vi "Main FPGA 5-axis for Candy Packaging.vi"() -> ()   [LabVIEW 2014]
uses:
  <vilib>/Motion/MotorControl/_s/nism.interpretControlRegister.stateTransition.ctl
  SubVIs/Pulse Trigger.ctl
  <vilib>/Platform/TimedLoop/XDataNode/timing_clust.ctl
  <vilib>/Platform/TimedLoop/XDataNode/nitl_modes.ctl
  <vilib>/Platform/TimedLoop/XDataNode/wakeup.ctl
  <vilib>/Motion/MotorControl/_s/nism.digitalInputs.portA.ctl
  <vilib>/rvi/Emulation/niFpgaGetClockAttributes.vi
  <vilib>/rvi/Emulation/niFpgaSctlEmulationGetInTimedLoop.vi
  <vilib>/rvi/Emulation/niFpgaEmulationReportErrorSimple.vi
  Global FPGA.vi
  <vilib>/Motion/MotorControl/_s/nism.interpretControlRegister.indexed.vi
  <vilib>/rvi/Emulation/niFpgaProcessEmulError.vi
  <vilib>/Motion/MotorControl/_s/nism.mdo.read.positionLoopSyncData.vi
  <vilib>/Motion/MotorControl/_s/nism.mdo.read.splineData.vi
  <vilib>/Motion/MotorControl/_s/nism.generateStatusRegister.indexed.vi
  <vilib>/rvi/Emulation/niFpgaCriticalErrorInLSC.vi
  <vilib>/Motion/MotorControl/_s/nism.splineInterpolation.fxp.3.index.vi
  <vilib>/Motion/MotorControl/_s/nism.mdo.handler.indexed.vi
  <vilib>/Motion/MotorControl/_s/nism.digitalFilter.indexed.vi
  <vilib>/Motion/MotorControl/_s/nism.interpretDIOControl.portA.multiple.vi
  <vilib>/Motion/MotorControl/_s/nism.generateDIOStatus.portA.indexed.2.vi
  <vilib>/rvi/eio/common/nirviEmuTemplateMethod_errors.vi
  <vilib>/Motion/SoftMotion/Synchronization/nism.rioScan.generateSyncScan.vi
  <vilib>/rvi/Emulation/niFpgaEmulationIsFPGAContextNoSignature.vi
  <vilib>/rvi/FIFO/Fifo_Resource/nirvififoEmulationSetSize.vi
  <vilib>/rvi/DataTransferAndStorage/Container/Common/niFpgaContainerGetUniqueNameForEmu.vi
  <vilib>/rvi/FIFO/Fifo_Resource/nirviFifoEmulationQueueMgr.vi
  <instcachedir>/0/nirviFifoEmulationQueueMgr_E5CAEC123FF24DC58D834DCA3CDAA9B5.lvgen/nirviFifoEmulationQueueMgr_E5CAEC123FF24DC58D834DCA3CDAA9B5_004.vi
  <vilib>/rvi/errors/niFpgaSetErrorForExecOnDevCompSimple.vi
  <vilib>/rvi/eio/common/nirviEmuReportErrorAndStop.vi
  <vilib>/rvi/FIFO/Fifo_Resource/nirvififoEmulationDetermineInputValidOut.vi
  <vilib>/rvi/FIFO/Fifo_Resource/nirvififoEmulationCreateLock.vi
  <vilib>/rvi/FIFO/Fifo_Resource/nirvififoEmulationObtainLock.vi
  <vilib>/rvi/FIFO/Fifo_Resource/nirvififoEmulationReleaseLock.vi
  <vilib>/rvi/occurrence/nirviWaitOnOccurrenceBase.vi
  <vilib>/rvi/errors/nirviReportUnexpectedCaseInternalError.vi
  <vilib>/rvi/errors/nirviReportUnexpectedCaseInternalError (U32).vi
  <vilib>/eio/EIONode/EIONode.xnode
  <vilib>/Platform/TimedLoop/XDataNode/XDataNode.xnode
  <vilib>/rvi/DataTransferAndStorage/Container/XNode/niFpgaContainer.xnode
  <vilib>/rvi/FIFO/Fifo_Resource/nirvififoEmulationClear.vi
  <vilib>/rvi/FIFO/Fifo_Resource/nirvififoEmulationGetNumberOfElementsToRead.vi
  <vilib>/rvi/FIFO/Fifo_Resource/nirvififoEmulationWrite.vi
  <vilib>/Motion/MotorControl/NI_SoftMotion_MotorControlIP.lvlib
  <vilib>/Platform/TimedLoop/XDataNode/XDNodeRunTimeDep.lvlib
  <vilib>/Motion/SoftMotion/Synchronization/NI_SoftMotion_Synchronization.lvlib
panel:
  in  "Mark Sensor Simulation":bool
  out "FIFO Elements to Read":u32
  in  "Use sim?":bool=TRUE
  out "Mod3/DIO0":bool
  out "TPeriod (ticks)":u32
  in  "TPulse (ticks)":i32=2000
  in  "Ta (ticks)":i32
  in  "Tb (ticks)":i32
  in  "Number of pulses (N)":i32=4
  out "FIFO Write Timed Out?":bool
  out "Remainder (ticks)":i32
  out "Processed Pulse":i32[](array[numeric])
  out "Ta Error":bool
  out "Tb Error":bool
  out "Tpulse Error":bool
  in  "Process Engine Mode":enum16{"Auto Calc Tpulse", "Auto Calc Tb"}(ring)
  in  "Reset?":bool
  in  "Clear FIFO":bool
  out "Reset Flag":bool
  in  "TDelay (ticks)":i32
  out "Process Engine State":T1
  out "Armed":bool
  in  "Axis 5 Mode":enum16{"No Sync", "Sync with Sensor"}(ring)
  in  "Sensor Sync DIR":bool
  out "FIFO Read Timed Out?":bool
  out "Time elapsed (ticks)":u32
  out "Toggle Iterations":u32
  in  "Home 5":bool
  in  "Home 4":bool
  in  "Home 3":bool
  in  "Home 2":bool
  in  "Home 1":bool
  out "Home Limits":bool[](array[boolean])
  out "Fwd Limits":bool[](array[boolean])
  out "Rev Limits":bool[](array[boolean])
  out "Axis Positions":fxp<+/-,64,32>[](array[numeric])
  in  "STEP or CW? (T=STEP)":bool
  out "Drive Enable":bool[](array[boolean])
  in  "Enable Watchdog":bool
  in  "Pet Watchdog":bool
  in  "Watchdog Timeout Period (ticks)":u64=40000000 format="%.0p"
  out "Watchdog Timed Out?":bool
  out "Time Since Last Pet":u64
  in  "Enable value":bool
  in  "Drive Enable override?":bool
  out "State":T2=enum."Start --> Initializing" caption="state transition"
  in  "Sync Value":bool
  in  "Sync Enable override?":bool
  in  "Invert direction?":bool
  out "Sync is Fault":bool
  out "Sync is Locked":bool
  in  "minimum pulse":u16=40
  # "Synchronization Loop"
  # "Control Status Loop"
  # "Notes: \n1. This VI provides the communication interface between the NI SoftMotion Engine and the LabVIEW FPGA Module. You must compile this VI for a specific FPGA target before use. After compiling, run the VI before running any of the Express VI examples. For information on moving this example to another FPGA target, refer to ni.com/info and enter info code fpgaex.\n\n2. Only use the Reset Axis button if you are unable to communicate with the axis by any other means. This button resets the device state machine and other VIs to a known state. After resetting the axis, switch the NI Scan Engine from Active Mode to Configuration Mode, then back to Active Mode, before attempting to enable the axis."
  # "(These two buttons \nare for testing\npurposes.)"
  # "(These two buttons \nare for testing\npurposes.)"
  # "Step/Direction Loop"
  # "Mark Sensor Sync Options"
  # "FIFO Check"
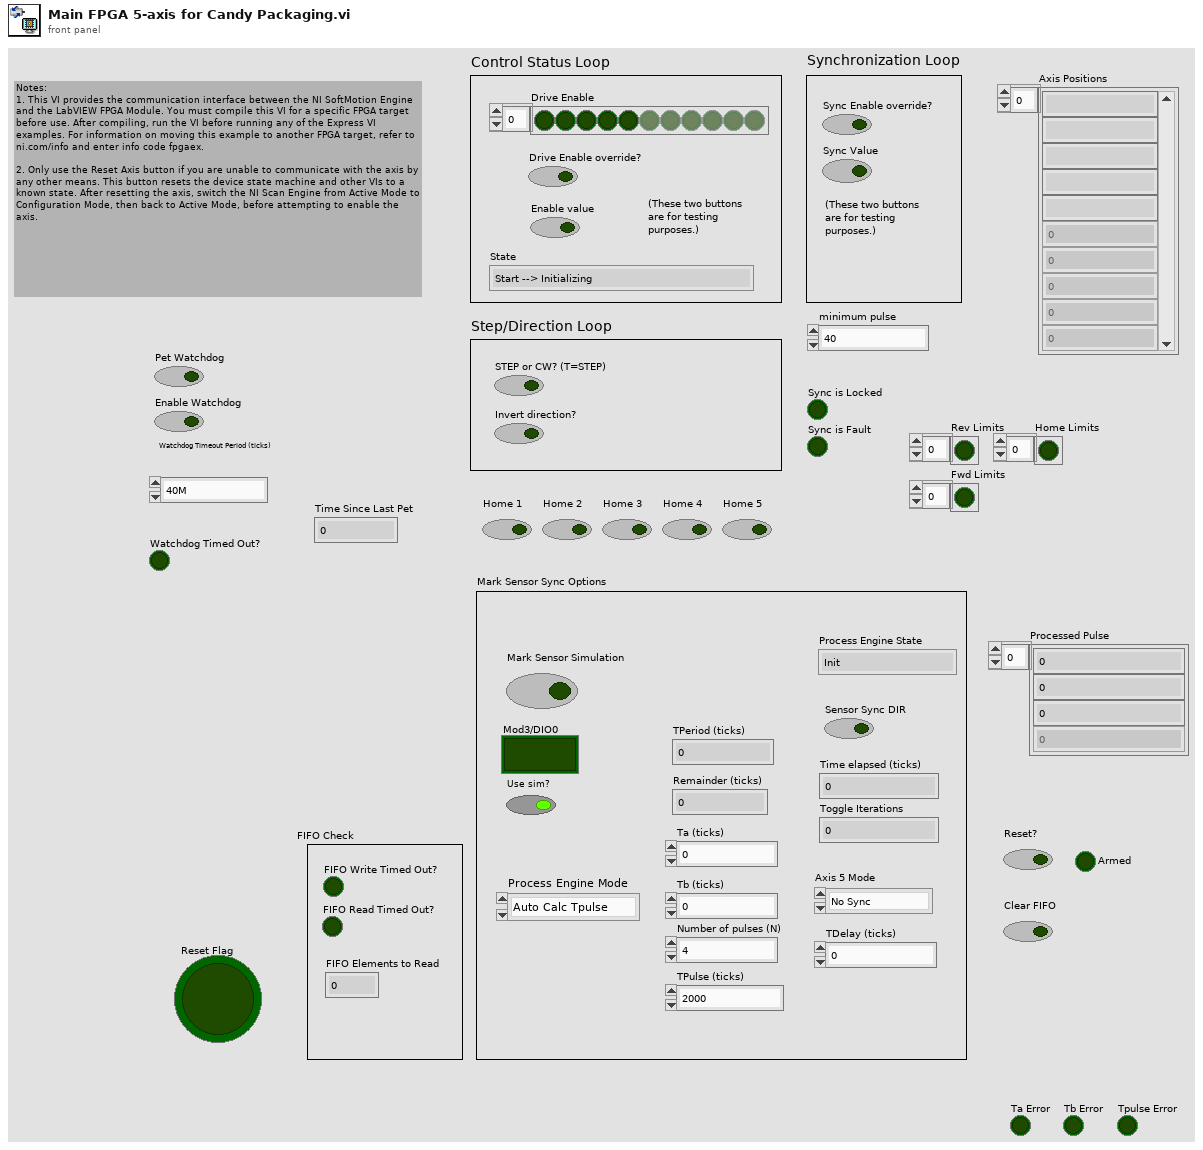
[diagram p1: front panel]
types:
  T1 = typedef "Pulse Trigger.ctl" = enum16{"Init", "Armed", "Processing"}
  T2 = typedef "NI_SoftMotion_MotorControlIP.lvlib/nism.interpretControlRegister.stateTransition.ctl" = enum8{"Invalid", "Start --> Initializing", "Initializing --> Disabled", "Disabled --> Ready To Switch On", "Ready To Switch On --> Switched On", "Ready To Switch On --> Disable", "Switched On --> Operation Enable", "Switched On --> Ready To Switch On", "Switched On --> Disabled", "Operation Enable --> Switched On", "Operation Enable --> Ready To Switch On", "Operation Enable --> Disabled", "Fault --> Disabled", "Any --> Fault", "None"}
  T3 = typedef "NI_SoftMotion_Synchronization.lvlib/nism.softmotionScan.timerConfig.ctl" = cluster{"target period (clocks)":u16, "host period / target period":u16}
  T4 = typedef "NI_SoftMotion_MotorControlIP.lvlib/nism.mdo.splineData.ctl" = cluster{"spline type":T5, "traj per/spline per":u16, "spline per/traj per":fxp<+,32,0>}
  T5 = typedef "NI_SoftMotion_MotorControlIP.lvlib/nism.splineInterpolation.type.ctl" = u16
  T6 = typedef "XDNodeRunTimeDep.lvlib/timing_clust.ctl" = cluster{"Expected End [f-1]":u64, "Actual End [f-1]":u64, "Finished Late? [f-1]":bool, "Expected End [i-1]":u64, "Actual End [i-1]":u64, "Finished Late? [i-1]":bool, "Expected Start [i]":u64, "Actual Start [i]":u64, "Expected Start [f]":u64, "Actual Start [f]":u64, "Source Name":string, "Structure Name":string, "Period":i64, "Deadline":i64, "Offset":i64, "Start":i64, "Priority":i32, "Timeout":i32, "Mode":T7, "Wakeup Reason":T8, "Error":errorcluster, "Source Type":string, "Secondary Source Type":string, "Global End Time":u64, "Global Start Time":u64, "Frame Duration":u64, "Iteration Duration":u64, "Assigned CPU":i32, "I/O Scan Engine Mode":u32}
  T7 = typedef "XDNodeRunTimeDep.lvlib/nitl_modes.ctl" = enum32{"No Change", "Process missed periods, maintain original phase", "Discard missed periods, maintain original phase", "Process missed periods, ignore original phase", "Discard missed periods, ignore original phase"}
  T8 = typedef "XDNodeRunTimeDep.lvlib/wakeup.ctl" = enum32{"Normal", "Aborted", "Asynchronous wakeup", "Timing source error", "Timed loop error", "Timeout"}
  T9 = typedef "NI_SoftMotion_Synchronization.lvlib/nism.softmotionScan.timerControl.ctl" = cluster{"sm scan":bool, "sm scan count":u32, "sm scan enabled":bool}
  T10 = typedef "NI_SoftMotion_MotorControlIP.lvlib/nism.digitalInputs.portA.ctl" = cluster{"reverse limit":bool, "forward limit":bool, "home switch":bool, "digital input 0":bool, "digital input 1":bool, "digital input 2":bool, "digital input 3":bool}
  T11 = typedef "NI_SoftMotion_MotorControlIP.lvlib/nism.dio.portA.config.2.ctl" = cluster{"digital filter (us)":u16[], "safe state":T12[]}
  T12 = typedef "nism.safeStates.ctl" = enum8{"Low", "High", "No Change"}
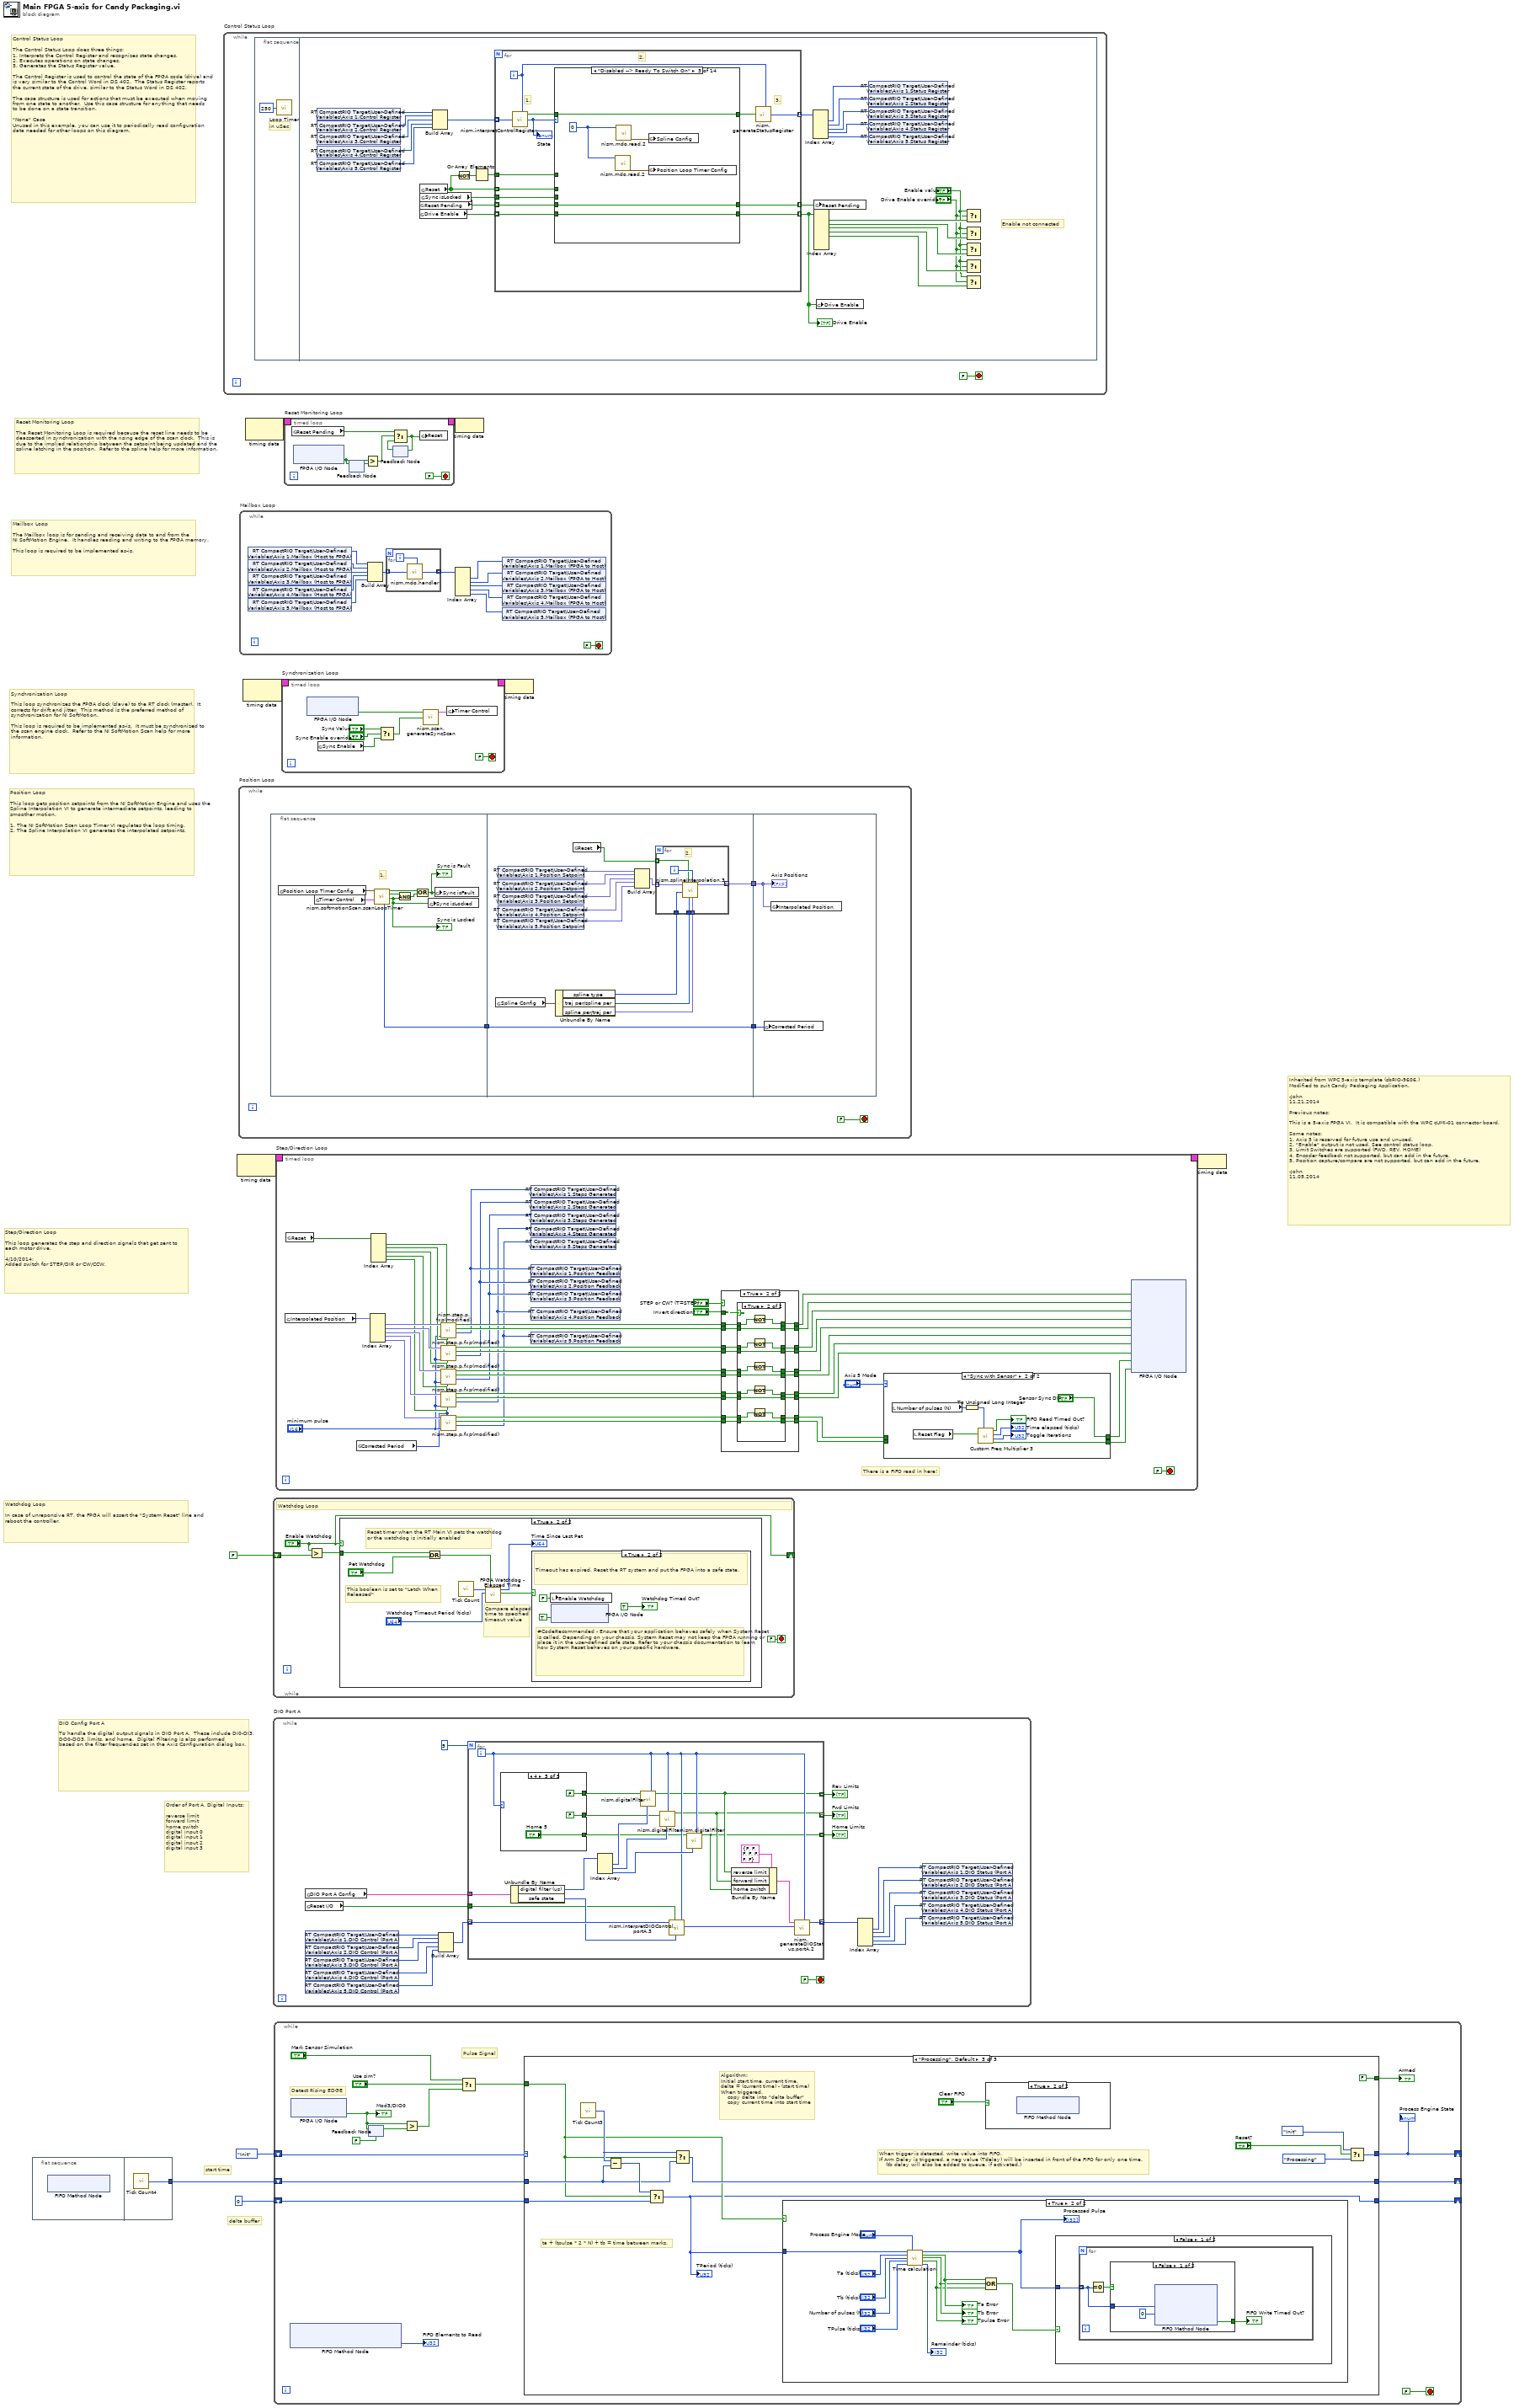
[diagram p0: block diagram]
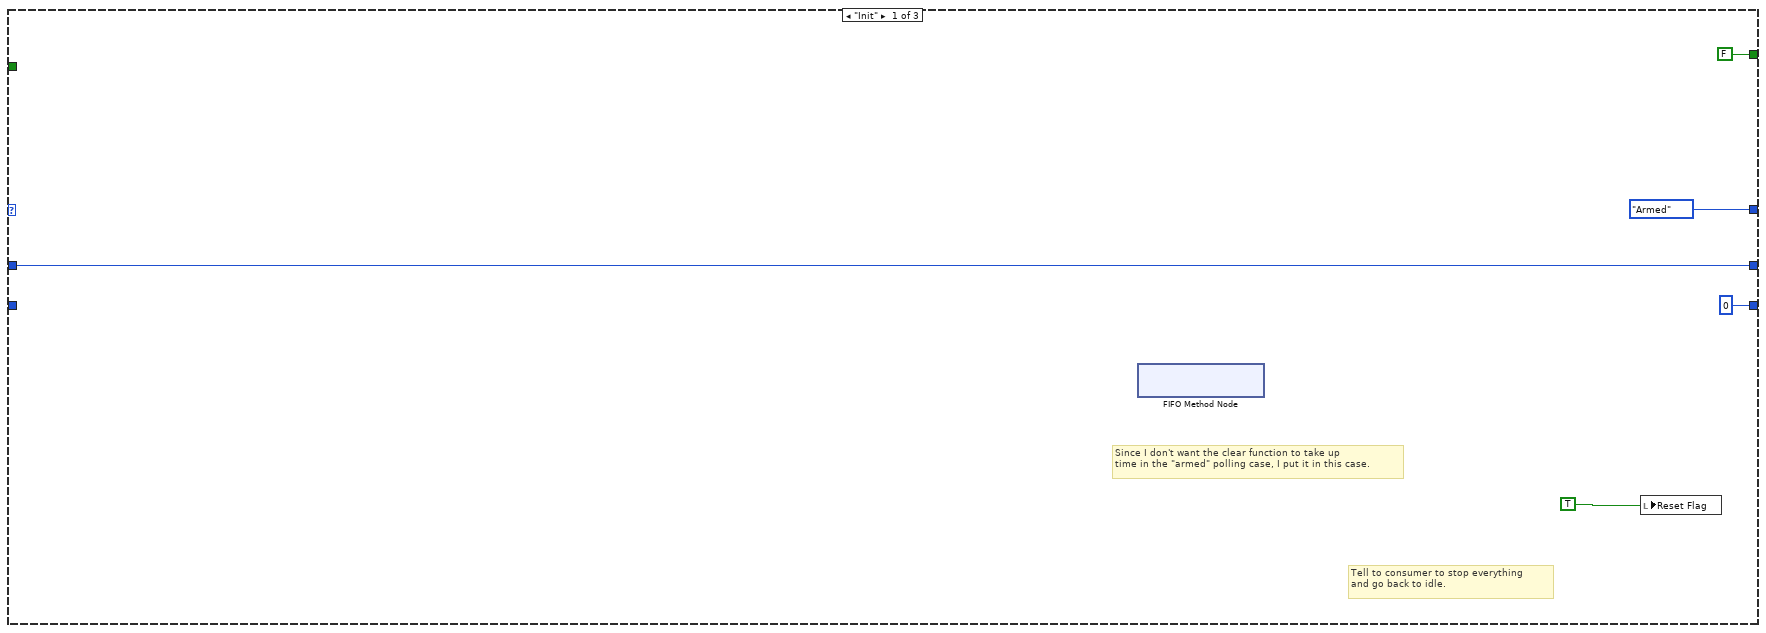
[diagram p2: hidden frame]
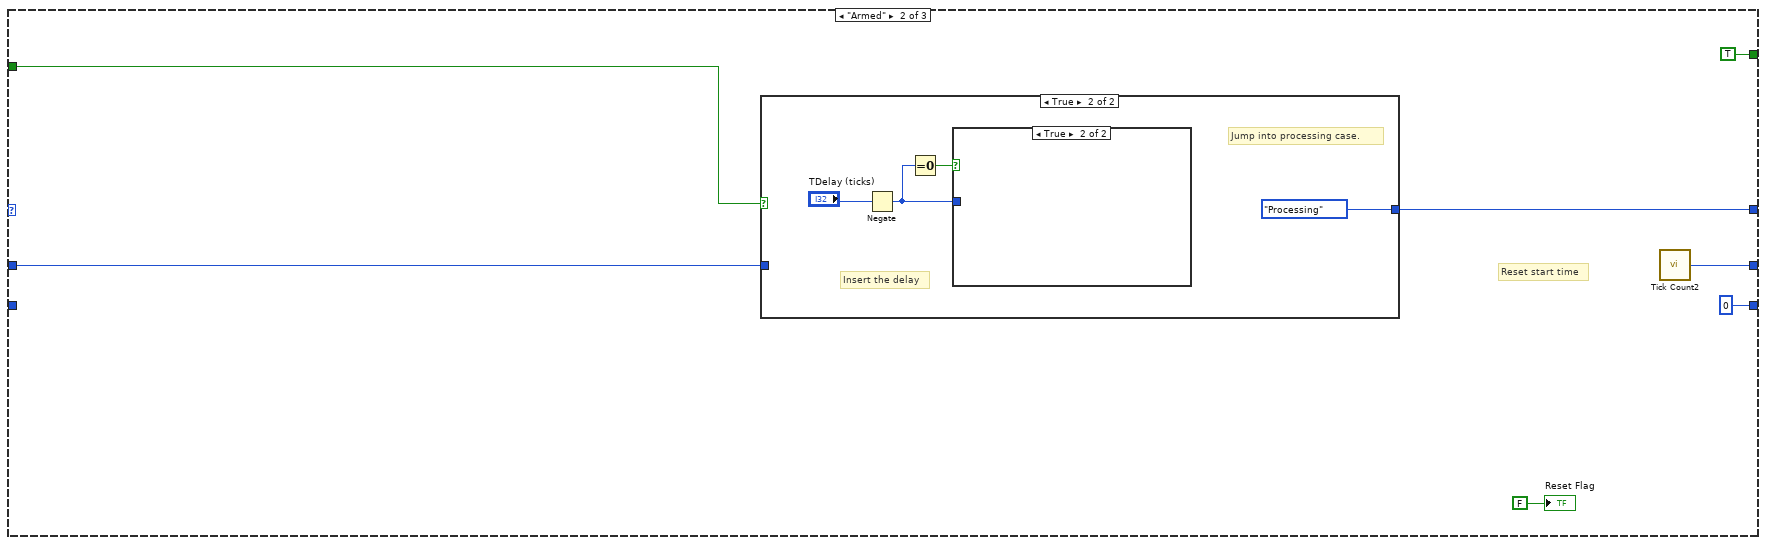
[diagram p3: hidden frame]
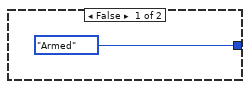
[diagram p4: hidden frame]
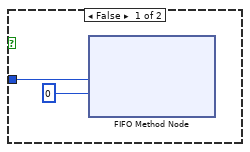
[diagram p5: hidden frame]
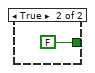
[diagram p8: hidden frame]
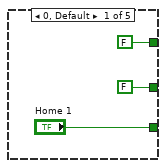
[diagram p10: hidden frame]
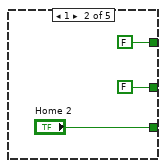
[diagram p11: hidden frame]
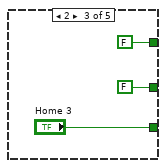
[diagram p12: hidden frame]
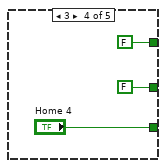
[diagram p13: hidden frame]
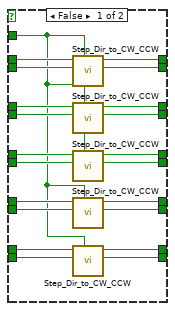
[diagram p17: hidden frame]
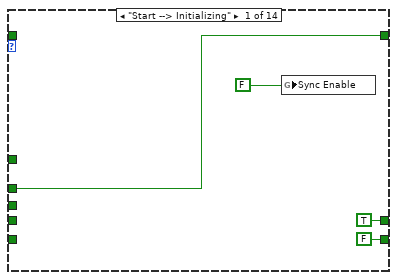
[diagram p19: hidden frame]
diagram:
  # "delta buffer"
  # "start time"
  # "Inherited from WPC 5-axis template (sbRIO-9606.)\nModified to suit Candy Packaging Application.\n\n-John\n11.21.2014\n\nPrevious notes:\n\nThis is a 5-axis FPGA VI.  It is compatible with the WPC cUMI-01 connector board.\n\nSome notes:\n1. Axis 5 is reserved for future use and unused.\n2. \"Enable\" output is not used. See control status loop.\n3. Limit Switches are supported (FWD, REV, HOME)\n4. Encoder feedback not supported, but can add in the future.\n5. Position capture/compare are not supported, but can add in the future.\n\n-John\n11.05.2014"
  # "DIO Config Port A\n\nTo handle the digital output signals in DIO Port A.  These include DI0-DI3, DO0-DO3, limits, and home.  Digital Filtering is also performed\nbased on the filter frequencies set in the Axis Configuration dialog box."
  # "Order of Port A, Digital Inputs:\n\nreverse limit\nforward limit\nhome switch\ndigital input 0\ndigital input 1\ndigital input 2\ndigital input 3"
  # "Watchdog Loop\n\nIn case of unreponsive RT, the FPGA will assert the \"System Reset\" line and reboot the controller."
  # "Step/Direction Loop\n\nThis loop generates the step and direction signals that get sent to \neach motor drive.\n\n4/10/2014:\nAdded switch for STEP/DIR or CW/CCW."
  # "Position Loop\n\nThis loop gets position setpoints from the NI SoftMotion Engine and uses the Spline Interpolation VI to generate intermediate setpoints, leading to smoother motion.\n\n1. The NI SoftMotion Scan Loop Timer VI regulates the loop timing. \n2. The Spline Interpolation VI generates the interpolated setpoints."
  # "Synchronization Loop\n\nThis loop synchronizes the FPGA clock (slave) to the RT clock (master).  It corrects for drift and jitter.  This method is the preferred method of synchronization for NI SoftMotion.\n\nThis loop is required to be implemented as-is.  It must be synchronized to the scan engine clock.  Refer to the NI SoftMotion Scan help for more information."
  # "Mailbox Loop\n\nThe Mailbox loop is for sending and receiving data to and from the \nNI SoftMotion Engine.  It handles reading and writing to the FPGA memory.\n\nThis loop is required to be implemented as-is."
  # "Reset Monitoring Loop\n\nThe Reset Monitoring Loop is required because the reset line needs to be deasserted in synchronization with the rising edge of the scan clock.  This is due to the implied relationship between the setpoint being updated and the spline latching in the position.  Refer to the spline help for more information."
  # "Control Status Loop\n\nThe Control Status Loop does three things:\n1. Interprets the Control Register and recognizes state changes.\n2. Executes operations on state changes.\n3. Generates the Status Register value.\n\nThe Control Register is used to control the state of the FPGA code (drive) and is very similar to the Control Word in DS 402.  The Status Register reports the current state of the drive, similar to the Status Word in DS 402.\n\nThe case structure is used for actions that must be executed when moving from one state to another.  Use this case structure for anything that needs to be done on a state transition.\n\n\"None\" Case\nUnused in this example, you can use it to periodically read configuration data needed for other loops on this diagram."
  n1 = flat-sequence {
    tunnel: [w11] -> w2
    frame #0 {
      n2 = xnode ("FIFO Method Node")() -> ()  [unwired: 1 in, 1 out]
    }
    frame #1 {
      n3 = call "Tick Count4"() -> ("Tick Count(Ticks)"=w11:u32)
    }
  }
  n4 = while "Control Status Loop" {
    stop <- FALSE stop-if-true
    n5 = flat-sequence {
      frame #0 {
        # "in uSec"
        n6 = call "Loop Timer"("Count(uSec)"=u32 250) -> ()  [unwired: 1 out]
      }
      frame #1 {
        # "Enable not connected"
        n7 = shared-variable "RT CompactRIO Target\\User-Defined Variables\\Axis 1.Control Register"() -> (w30:u32)  [unwired: 1 in, 1 out]
        n8 = shared-variable "RT CompactRIO Target\\User-Defined Variables\\Axis 2.Control Register"() -> (w29:u32)  [unwired: 1 in, 1 out]
        n9 = shared-variable "RT CompactRIO Target\\User-Defined Variables\\Axis 3.Control Register"() -> (w28:u32)  [unwired: 1 in, 1 out]
        n10 = shared-variable "RT CompactRIO Target\\User-Defined Variables\\Axis 4.Control Register"() -> (w27:u32)  [unwired: 1 in, 1 out]
        n11 = shared-variable "RT CompactRIO Target\\User-Defined Variables\\Axis 5.Control Register"() -> (w26:u32)  [unwired: 1 in, 1 out]
        n12 = global read "Global FPGA.vi" "Reset Pending"() -> (w34:bool[])
        n13 = global read "Global FPGA.vi" "Drive Enable"() -> (w33:bool[])
        n14 = global read "Global FPGA.vi" "Reset"() -> (w35:bool[])
        n15 = global read "Global FPGA.vi" "Sync isLocked"() -> (w40:bool)
        n16 = Build Array(w30, w29, w28, w27, w26) -> (w39:u32[])
        n17 = Not(x=w35) -> (.not. x?=w37:bool[])
        n18 = Or Array Elements(Boolean array=w37) -> (logical OR=w36:bool)
        n19 = for {
          tunnel: w35 -> [w48] mode=indexing
          tunnel: w40 -> [w47]
          tunnel: w39 -> [w49] mode=indexing
          tunnel: [w46] -> w31 mode=indexing
          tunnel: [w45] -> w38 mode=indexing
          tunnel: [w44] -> w32 mode=indexing
          tunnel: w36 -> [w43]
          tunnel: w34 -> [w42] mode=indexing
          tunnel: w33 -> [w41] mode=indexing
          i -> [w50]
          # "3."
          # "2."
          # "1."
          n20 = call-poly <vilib>:"nism.interpretControlRegister.vi"("control register"=w49, "axis index"=w50) -> ("transition occurred"=w51:bool, "state transition"=w52:T2)  [unwired: 6 in]
          "State" <- w52
          n21 = case shown="\"Disabled --> Ready To Switch On\"" w52 {
            tunnel: w51 -> [_ w60 w66 _ w73 _ w81 w85 _ _ _ _ w105 _]
            tunnel: [w57 w60 w66 w68 w73 w77 w81 w85 w87 w90 w94 w98 w104 _] -> w53
            tunnel: w48 -> [w57 _ _ _ _ w76 _ _ w87 w90 w94 w98 _ _]
            tunnel: w47 -> [_ _ _ w68 _ _ _ _ _ _ _ _ _ _]
            tunnel: [TRUE ("Write.Reset Pending") w59 w63 w67 w72 FALSE ("Write.Reset Pending") w78 w82 TRUE ("Write.Reset Pending") TRUE ("Write.Reset Pending") TRUE ("Write.Reset Pending") TRUE ("Write.Reset Pending") w102 w107] -> w45
            tunnel: [FALSE ("Write.Drive Enable") w58 w62 TRUE ("Write.Drive Enable") w71 w74 FALSE ("Write.Drive Enable") FALSE ("Write.Drive Enable") w86 FALSE ("Write.Drive Enable") FALSE ("Write.Drive Enable") FALSE ("Write.Drive Enable") w101 w106] -> w44
            tunnel: w43 -> [_ _ _ _ _ _ w79 w83 _ w89 w93 w97 w103 _]
            tunnel: w42 -> [_ w59 w63 w67 w72 _ w78 w82 _ _ _ _ w102 w107]
            tunnel: w41 -> [_ w58 w62 _ w71 w74 _ _ w86 _ _ _ w101 w106]
            frame "Start --> Initializing" {
              n22 = global write "Global FPGA.vi" "Sync Enable"(FALSE ("Sync Enable")) -> ()
            }
            frame "Initializing --> Disabled" {
            }
            frame "Disabled --> Ready To Switch On" {
              w61 = 0 ("axis index")
              n23 = call-poly <vilib>:"nism.mdo.read.2.vi"("axis index"=w61) -> ("position loop sync"=w64:T3)  [unwired: 10 in]
              n24 = call-poly <vilib>:"nism.mdo.read.2.vi"("axis index"=w61) -> ("spline"=w65:T4)  [unwired: 10 in]
              n25 = global write "Global FPGA.vi" "Spline Config"(w65) -> ()
              n26 = global write "Global FPGA.vi" "Position Loop Timer Config"(w64) -> ()
            }
            frame "Ready To Switch On --> Switched On" {
              n27 = global write "Global FPGA.vi" "Sync Enable"(TRUE ("Sync Enable")) -> ()
            }
            frame "Ready To Switch On --> Disable" {
            }
            frame "Switched On --> Operation Enable" {
              n28 = Not(x=w76) -> (.not. x?=w77:bool)
            }
            frame "Switched On --> Ready To Switch On" {
              n29 = global write "Global FPGA.vi" "Sync Enable"(w79) -> ()
            }
            frame "Switched On --> Disabled" {
              n30 = global write "Global FPGA.vi" "Sync Enable"(w83) -> ()
            }
            frame "Operation Enable --> Switched On" {
            }
            frame "Operation Enable --> Ready To Switch On" {
              n31 = global write "Global FPGA.vi" "Sync Enable"(w89) -> ()
            }
            frame "Operation Enable --> Disabled" {
              n32 = global write "Global FPGA.vi" "Sync Enable"(w93) -> ()
            }
            frame "Any --> Fault" {
              n33 = global write "Global FPGA.vi" "Sync Enable"(w97) -> ()
            }
            frame "Fault --> Disabled" {
              # "wait one cycle for clear faults to have taken effect"
              n34 = global write "Global FPGA.vi" "Sync Enable"(w103) -> ()
              n35 = Not(x=w105) -> (.not. x?=w104:bool)
            }
            frame "None", Default {
            }
          }
          n36 = call-poly <vilib>:"nism.generateStatusRegister.vi"("transition success"=w53, "axis index"=w50) -> ("status register"=w46:u32)  [unwired: 7 in]
        }
        "Drive Enable" <- w32
        n37 = Index Array(array=w31) -> (element #1=w25:u32, element #2=w24:u32, element #3=w23:u32, element #4=w22:u32, element #5=w21:u32)  [unwired: 5 in]
        n38 = global write "Global FPGA.vi" "Reset Pending"(w38) -> ()
        n39 = Index Array(array=w32) -> (element #1=w20:bool, element #2=w19:bool, element #3=w18:bool, element #4=w17:bool, element #5=w16:bool)  [unwired: 8 in, 3 out]
        n40 = global write "Global FPGA.vi" "Drive Enable"(w32) -> ()
        n41 = shared-variable "RT CompactRIO Target\\User-Defined Variables\\Axis 1.Status Register"(w25) -> ()  [unwired: 1 in, 1 out]
        n42 = shared-variable "RT CompactRIO Target\\User-Defined Variables\\Axis 2.Status Register"(w24) -> ()  [unwired: 1 in, 1 out]
        n43 = shared-variable "RT CompactRIO Target\\User-Defined Variables\\Axis 3.Status Register"(w23) -> ()  [unwired: 1 in, 1 out]
        n44 = shared-variable "RT CompactRIO Target\\User-Defined Variables\\Axis 4.Status Register"(w22) -> ()  [unwired: 1 in, 1 out]
        n45 = shared-variable "RT CompactRIO Target\\User-Defined Variables\\Axis 5.Status Register"(w21) -> ()  [unwired: 1 in, 1 out]
        n46 = Select(t="Enable value", s="Drive Enable override?", f=w20) -> ()  [unwired: 1 out]
        n47 = Select(t="Enable value", s="Drive Enable override?", f=w19) -> ()  [unwired: 1 out]
        n48 = Select(t="Enable value", s="Drive Enable override?", f=w18) -> ()  [unwired: 1 out]
        n49 = Select(t="Enable value", s="Drive Enable override?", f=w17) -> ()  [unwired: 1 out]
        n50 = Select(t="Enable value", s="Drive Enable override?", f=w16) -> ()  [unwired: 1 out]
      }
    }
  }
  n51 = node-c288() -> (w10:T6)  [unwired: 1 in]
  n52 = while "Position Loop" {
    stop <- FALSE stop-if-true
    n53 = flat-sequence {
      tunnel: [w112] -> w108
      tunnel: [w126] -> w110
      tunnel: [w125] -> w109
      tunnel: w108 -> [w125]
      tunnel: w110 -> [w140]
      tunnel: w109 -> [w141]
      frame #0 {
        # "1."
        n54 = global read "Global FPGA.vi" "Position Loop Timer Config"() -> (w114:T3)
        n55 = global read "Global FPGA.vi" "Timer Control"() -> (w113:T9)
        n56 = call <vilib>:"nism.softmotionScan.scanLoopTimer.vi"("timer control"=w113, "timer config"=w114) -> ("scan running?"=w116:bool, "finished late?"=w118:bool, "fault occurred?"=w119:bool, "corrected period"=w112:u16)  [unwired: 5 in, 1 out]
        "Sync is Locked" <- w116
        n57 = Compound Arithmetic op=AND(w118, w116) -> (w117:bool)
        n58 = Compound Arithmetic op=OR(w119, w117) -> (w115:bool)
        "Sync is Fault" <- w115
        n59 = global write "Global FPGA.vi" "Sync isLocked"(w116) -> ()
        n60 = global write "Global FPGA.vi" "Sync isFault"(w115) -> ()
      }
      frame #1 {
        n61 = global read "Global FPGA.vi" "Spline Config"() -> (w128:T4)
        n62 = shared-variable "RT CompactRIO Target\\User-Defined Variables\\Axis 1.Position Setpoint"() -> (w124:fxp<+/-,64,32>)  [unwired: 1 in, 1 out]
        n63 = shared-variable "RT CompactRIO Target\\User-Defined Variables\\Axis 2.Position Setpoint"() -> (w123:fxp<+/-,64,32>)  [unwired: 1 in, 1 out]
        n64 = shared-variable "RT CompactRIO Target\\User-Defined Variables\\Axis 3.Position Setpoint"() -> (w122:fxp<+/-,64,32>)  [unwired: 1 in, 1 out]
        n65 = shared-variable "RT CompactRIO Target\\User-Defined Variables\\Axis 4.Position Setpoint"() -> (w121:fxp<+/-,64,32>)  [unwired: 1 in, 1 out]
        n66 = shared-variable "RT CompactRIO Target\\User-Defined Variables\\Axis 5.Position Setpoint"() -> (w120:fxp<+/-,64,32>)  [unwired: 1 in, 1 out]
        n67 = Unbundle By Name(w128) -> ("spline type"=w132:T5, "traj per/spline per"=w131:u16, "spline per/traj per"=w130:fxp<+,32,0>)
        n68 = global read "Global FPGA.vi" "Reset"() -> (w127:bool[])
        n69 = Build Array(w124, w123, w122, w121, w120) -> (w129:fxp<+/-,64,32>[])
        n70 = for {
          tunnel: w132 -> [w139]
          tunnel: w131 -> [w138]
          tunnel: w130 -> [w137]
          tunnel: w127 -> [w134] mode=indexing
          tunnel: w129 -> [w136] mode=indexing
          tunnel: [w133] -> w126 mode=indexing
          i -> [w135]
          # "2."
          n71 = call-poly <vilib>:"nism.splineInterpolation.3.vi"("1 / calls per sample"=w137, "index"=w135, "calls per sample"=w138, "reset"=w134, "spline type"=w139, "x"=w136) -> ("xi"=w133:fxp<+/-,64,32>)  [unwired: 4 in, 1 out]
        }
      }
      frame #2 {
        n72 = global write "Global FPGA.vi" "Corrected Period"(w141) -> ()
        n73 = global write "Global FPGA.vi" "Interpolated Position"(w140) -> ()
        "Axis Positions" <- w140
      }
    }
  }
  n74 = while "Mailbox Loop" {
    stop <- FALSE stop-if-true
    n75 = shared-variable "RT CompactRIO Target\\User-Defined Variables\\Axis 1.Mailbox (Host to FPGA)"() -> (w151:u64)  [unwired: 1 in, 1 out]
    n76 = shared-variable "RT CompactRIO Target\\User-Defined Variables\\Axis 2.Mailbox (Host to FPGA)"() -> (w150:u64)  [unwired: 1 in, 1 out]
    n77 = shared-variable "RT CompactRIO Target\\User-Defined Variables\\Axis 3.Mailbox (Host to FPGA)"() -> (w149:u64)  [unwired: 1 in, 1 out]
    n78 = shared-variable "RT CompactRIO Target\\User-Defined Variables\\Axis 4.Mailbox (Host to FPGA)"() -> (w148:u64)  [unwired: 1 in, 1 out]
    n79 = shared-variable "RT CompactRIO Target\\User-Defined Variables\\Axis 5.Mailbox (Host to FPGA)"() -> (w147:u64)  [unwired: 1 in, 1 out]
    n80 = Build Array(w151, w150, w149, w148, w147) -> (w153:u64[])
    n81 = for {
      tunnel: w153 -> [w157] mode=indexing
      tunnel: [w156] -> w152 mode=indexing
      i -> [w155]
      n82 = call-poly <vilib>:"nism.mdo.handler.vi"("mbox (host to fpga)"=w157, "axis index"=w155) -> ("mbox (fpga to host)"=w156:u64)  [unwired: 7 in]
    }
    n83 = Index Array(array=w152) -> (element #1=w146:u64, element #2=w145:u64, element #3=w144:u64, element #4=w143:u64, element #5=w142:u64)  [unwired: 5 in]
    n84 = shared-variable "RT CompactRIO Target\\User-Defined Variables\\Axis 5.Mailbox (FPGA to Host)"(w142) -> ()  [unwired: 1 in, 1 out]
    n85 = shared-variable "RT CompactRIO Target\\User-Defined Variables\\Axis 1.Mailbox (FPGA to Host)"(w146) -> ()  [unwired: 1 in, 1 out]
    n86 = shared-variable "RT CompactRIO Target\\User-Defined Variables\\Axis 2.Mailbox (FPGA to Host)"(w145) -> ()  [unwired: 1 in, 1 out]
    n87 = shared-variable "RT CompactRIO Target\\User-Defined Variables\\Axis 3.Mailbox (FPGA to Host)"(w144) -> ()  [unwired: 1 in, 1 out]
    n88 = shared-variable "RT CompactRIO Target\\User-Defined Variables\\Axis 4.Mailbox (FPGA to Host)"(w143) -> ()  [unwired: 1 in, 1 out]
  }
  n89 = node-c288() -> (w8:T6)  [unwired: 1 in]
  n90 = node-c288() -> (w6:T6)  [unwired: 1 in]
  n91 = while "RT Watchdog Loop" {
    shift-right: ["Enable Watchdog"] -> _
    shift-left: FALSE ("Enable RT Watchdog") -> [w161]
    stop <- FALSE stop-if-true
    # "Watchdog Loop"
    n92 = Greater?(x="Enable Watchdog", y=w161) -> (0:w158:bool)
    n93 = case shown="True" "Enable Watchdog" {
      tunnel: w158 -> [_ w164]
      frame False {
        # "This loop has to be explicitly enabled from the RT Main VI.  This reduces the possiblity of an endless reboot cycle."
      }
      frame True {
        # "This boolean is set to \"Latch When Released\""
        # "Compare elapsed time to specified timeout value"
        # "Reset timer when the RT Main VI pets the watchdog or the watchdog is initially enabled"
        n94 = Or(x=w164, y="Pet Watchdog") -> (x .or. y?=w163:bool)
        n95 = call "Tick Count"() -> ("Tick Count(Ticks)"=w167:u32)
        n96 = call "FPGA Watchdog - Elapsed Time.vi"("Reset"=w163, "Timeout Period"="Watchdog Timeout Period (ticks)", "Current Time"=w167) -> ("Timeout"=w162:bool, "Elapsed Time"=→"Time Since Last Pet":u64)  [unwired: 7 in]
        n97 = case shown="True" w162 {
          frame False {
            # "Timeout has not expired."
          }
          frame True {
            # "#CodeRecommended - Ensure that your application behaves safely when System Reset is called. Depending on your chassis, System Reset may not keep the FPGA running or place it in the user-defined safe state. Refer to your chassis documentation to learn how System Reset behaves on your specific hardware."
            # "Timeout has expired. Reset the RT system and put the FPGA into a safe state."
            n98 = local write "Enable Watchdog"(FALSE ("Enable RT Watchdog")) -> ()
            n99 = xnode "FPGA I/O Node"("System Reset"=TRUE ("RT Reset on Watchdog Failure?")) -> ()  [unwired: 1 in, 1 out]
            "Watchdog Timed Out?" <- TRUE ("Watchdog Timed Out?")
          }
        }
      }
    }
  }
  n100 = while "DIO Port A" {
    stop <- FALSE stop-if-true
    n101 = global read "Global FPGA.vi" "DIO Port A Config"() -> (w189:T11)
    n102 = global read "Global FPGA.vi" "Reset I/O"() -> (w188:bool)
    n103 = shared-variable "RT CompactRIO Target\\User-Defined Variables\\Axis 1.DIO Control (Port A)"() -> (w186:u32)  [unwired: 1 in, 1 out]
    n104 = shared-variable "RT CompactRIO Target\\User-Defined Variables\\Axis 2.DIO Control (Port A)"() -> (w185:u32)  [unwired: 1 in, 1 out]
    n105 = shared-variable "RT CompactRIO Target\\User-Defined Variables\\Axis 3.DIO Control (Port A)"() -> (w184:u32)  [unwired: 1 in, 1 out]
    n106 = shared-variable "RT CompactRIO Target\\User-Defined Variables\\Axis 4.DIO Control (Port A)"() -> (w183:u32)  [unwired: 1 in, 1 out]
    n107 = shared-variable "RT CompactRIO Target\\User-Defined Variables\\Axis 5.DIO Control (Port A)"() -> (w182:u32)  [unwired: 1 in, 1 out]
    n108 = Build Array(w186, w185, w184, w183, w182) -> (w181:u32[])
    n109 = for {
      N: 5 -> [_]
      tunnel: [w208] -> w175 mode=indexing
      tunnel: w181 -> [w207] mode=indexing
      tunnel: w189 -> [w204]
      tunnel: w188 -> [w202]
      tunnel: [w193] -> w174 mode=indexing
      tunnel: [w192] -> w173 mode=indexing
      tunnel: [w191] -> w172 mode=indexing
      i -> [w197]
      n110 = case shown="4" w197 {
        tunnel: [FALSE ("RMC/DIO44") FALSE ("RMC/DIO44") FALSE ("RMC/DIO44") FALSE ("RMC/DIO44") FALSE ("RMC/DIO44")] -> w196
        tunnel: ["Home 1" "Home 2" "Home 3" "Home 4" "Home 5"] -> w195
        tunnel: [FALSE ("RMC/DIO77") FALSE ("RMC/DIO77") FALSE ("RMC/DIO77") FALSE ("RMC/DIO77") FALSE ("RMC/DIO77")] -> w194
        frame 0, Default {
        }
        frame 1 {
        }
        frame 2 {
        }
        frame 3 {
        }
        frame 4 {
        }
      }
      n111 = Unbundle By Name(w204) -> ("digital filter (us)"=w198:u16[], "safe state"=w203:T12[])
      n112 = Index Array(array=w198) -> (element #1=w199:u16, element #2=w200:u16, element #3=w201:u16)  [unwired: 3 in]
      n113 = call-poly <vilib>:"nism.digitalFilter.vi"("index"=w197, "filter value (us)"=w199, "input signal"=w196) -> ("output signal"=w193:bool)  [unwired: 8 in]
      n114 = call-poly <vilib>:"nism.digitalFilter.vi"("index"=w197, "filter value (us)"=w200, "input signal"=w194) -> ("output signal"=w192:bool)  [unwired: 8 in]
      n115 = call-poly <vilib>:"nism.interpretDIOControl.portA.3.vi"("index"=w197, "safe state"=w203, "reset"=w202, "dio control(port a)"=w207) -> ("reset latches"=w209:u8)  [unwired: 6 in, 1 out]
      n116 = call-poly <vilib>:"nism.digitalFilter.vi"("index"=w197, "filter value (us)"=w201, "input signal"=w195) -> ("output signal"=w191:bool)  [unwired: 8 in]
      n117 = Bundle By Name(cluster=T10 {"reverse limit"=FALSE, "forward limit"=FALSE, "home switch"=FALSE, "digital input 0"=FALSE, "digital input 1"=FALSE, "digital input 2"=FALSE, "digital input 3"=FALSE} ("$(driveInterface.digitalInputs.shortName)"), "reverse limit"=w193, "forward limit"=w192, "home switch"=w191) -> (w205:T10)
      n118 = call-poly <vilib>:"nism.generateDIOStatus.portA.2.vi"("index"=w197, "reset latches"=w209, "digital inputs"=w205) -> ("dio status(port a)"=w208:u32)  [unwired: 8 in]
    }
    "Rev Limits" <- w174
    "Fwd Limits" <- w173
    "Home Limits" <- w172
    n119 = Index Array(array=w175) -> (element #1=w180:u32, element #2=w179:u32, element #3=w178:u32, element #4=w177:u32, element #5=w176:u32)  [unwired: 5 in]
    n120 = shared-variable "RT CompactRIO Target\\User-Defined Variables\\Axis 1.DIO Status (Port A)"(w180) -> ()  [unwired: 1 in, 1 out]
    n121 = shared-variable "RT CompactRIO Target\\User-Defined Variables\\Axis 2.DIO Status (Port A)"(w179) -> ()  [unwired: 1 in, 1 out]
    n122 = shared-variable "RT CompactRIO Target\\User-Defined Variables\\Axis 3.DIO Status (Port A)"(w178) -> ()  [unwired: 1 in, 1 out]
    n123 = shared-variable "RT CompactRIO Target\\User-Defined Variables\\Axis 4.DIO Status (Port A)"(w177) -> ()  [unwired: 1 in, 1 out]
    n124 = shared-variable "RT CompactRIO Target\\User-Defined Variables\\Axis 5.DIO Status (Port A)"(w176) -> ()  [unwired: 1 in, 1 out]
  }
  n125 = while {
    shift-right: [w238] -> _
    shift-left: w2 -> [w239]
    shift-right: [w232] -> _
    shift-left: u32 0 -> [w240]
    shift-right: [w226] -> _
    shift-left: Pulse_Trigger."Init" -> [w227]
    stop <- FALSE stop-if-true
    # "Pulse Signal"
    # "Detect Rising EDGE"
    n126 = xnode ("FIFO Method Node")() -> ("Number of Elements to Read"=→"FIFO Elements to Read":u32)  [unwired: 1 in, 1 out]
    n127 = xnode "FPGA I/O Node"() -> ("Mod3/DIO0"=w228:bool)  [unwired: 1 in, 1 out]
    "Mod3/DIO0" <- w228
    n128 = feedback-in #1(w228) -> ()
    n129 = feedback #1(FALSE) -> (w230:bool)
    n130 = Greater?(x=w228, y=w230) -> (0:w229:bool)
    n131 = Select(t="Mark Sensor Simulation", s="Use sim?", f=w229) -> (s? t:f=w233:bool)
    n132 = case shown="\"Processing\", Default" w227 {
      tunnel: w240 -> [_ _ w271]
      tunnel: w239 -> [w243 w248 w269]
      tunnel: [w243 w247 w268] -> w238
      tunnel: w233 -> [_ w250 w267]
      tunnel: [u32 0 u32 0 w262] -> w232
      tunnel: [Pulse_Trigger."Armed" w249 w264] -> w226
      tunnel: [FALSE ("Armed") TRUE ("Armed") FALSE ("Armed")] -> w225
      frame "Init" {
        # "Tell to consumer to stop everything \nand go back to idle."
        # "Since I don't want the clear function to take up\ntime in the \"armed\" polling case, I put it in this case."
        n133 = xnode ("FIFO Method Node")() -> ()  [unwired: 1 in, 1 out]
        n134 = local write "Reset Flag"(TRUE) -> ()
      }
      frame "Armed" {
        # "Reset start time"
        n135 = case shown="True" w250 {
          tunnel: [Pulse_Trigger."Armed" Pulse_Trigger."Processing"] -> w249
          tunnel: w248 -> [_ _]
          frame False {
          }
          frame True {
            # "Insert the delay"
            # "Jump into processing case."
            n136 = Negate(x="TDelay (ticks)") -> (-x=w254:i32)
            n137 = Equal To 0?(x=w254) -> (x = 0?=w255:bool)
            n138 = case shown="True" w255 {
              tunnel: w254 -> [w259 _]
              frame False {
                n139 = xnode ("FIFO Method Node")("Element"=w259, "Timeout"=0) -> ()  [unwired: 1 in, 2 out]
              }
              frame True {
              }
            }
          }
        }
        n140 = call "Tick Count2"() -> ("Tick Count(Ticks)"=w247:u32)
        "Reset Flag" <- FALSE ("Boolean")
      }
      frame "Processing", Default {
        # "ta + (tpulse * 2 * N) + tb = time between marks."
        # "When trigger is detected, write value into FIFO.\nIf Arm Delay is triggered, a neg value (Tdelay) will be inserted in front of the FIFO for only one time.\n    (tb delay will also be added to queue, if activated.)"
        # "Algorithm:\nInitial start time, current time.\ndelta = (current time) - (start time)\nWhen triggered,\n    copy delta into \"delta buffer\"\n    copy current time into start time"
        n141 = call "Tick Count3"() -> ("Tick Count(Ticks)"=w270:u32)
        n142 = Subtract(x=w270, y=w269) -> (x-y=w272:u32)
        n143 = Select(t=w272, s=w267, f=w271) -> (s? t:f=w262:u32)
        "TPeriod (ticks)" <- w262
        n144 = Select(t=w270, s=w267, f=w269) -> (s? t:f=w268:u32)
        n145 = case shown="True" w267 {
          tunnel: w262 -> [_ w284]
          frame False {
          }
          frame True {
            n146 = call "Time calculation.vi"("Time between marks (ticks)"=w284, "Mode"="Process Engine Mode", "Ta (ticks)"="Ta (ticks)", "Tb (ticks)"="Tb (ticks)", "Number of pulses (N)"="Number of pulses (N)", "TPulse (ticks)"="TPulse (ticks)") -> ("appended array"=w278:i32[], "Ta Error"=w277:bool, "Tb Error"=w276:bool, "Tpulse Error"=w275:bool, "Remainder (ticks)"=→"Remainder (ticks)":i32)  [unwired: 5 in]
            "Processed Pulse" <- w278
            "Ta Error" <- w277
            "Tb Error" <- w276
            "Tpulse Error" <- w275
            n147 = Compound Arithmetic op=OR(w277, w276, w275) -> (w274:bool)
            n148 = case shown="False" w274 {
              tunnel: w278 -> [w285 _]
              frame False {
                n149 = for {
                  tunnel: w285 -> [w287] mode=indexing
                  n150 = Equal To 0?(x=w287) -> (x = 0?=w288:bool)
                  n151 = case shown="False" w288 {
                    tunnel: [w290 FALSE ("Timed Out?")] -> w286
                    tunnel: w287 -> [w289 _]
                    frame False {
                      n152 = xnode ("FIFO Method Node")("Element"=w289, "Timeout"=0) -> ("Timed Out?"=w290:bool)  [unwired: 1 in, 1 out]
                    }
                    frame True {
                    }
                  }
                  "FIFO Write Timed Out?" <- w286
                }
              }
              frame True {
              }
            }
          }
        }
        n153 = case shown="True" "Clear FIFO" {
          frame False {
          }
          frame True {
            n154 = xnode ("FIFO Method Node")() -> ()  [unwired: 1 in, 1 out]
          }
        }
        n155 = Select(t=Pulse_Trigger."Init", s="Reset?", f=Pulse_Trigger."Processing") -> (s? t:f=w264:T1)
      }
    }
    "Process Engine State" <- w226
    "Armed" <- w225
  }
  n156 = timed-loop "Step/Direction Loop" {
    timing: w10 -> [_]
    timing-out: [_] -> w9
    stop <- FALSE stop-if-true
    # "There is a FIFO read in here!"
    n157 = global read "Global FPGA.vi" "Interpolated Position"() -> (w336:fxp<+/-,64,32>[])
    n158 = global read "Global FPGA.vi" "Reset"() -> (w330:bool[])
    n159 = global read "Global FPGA.vi" "Corrected Period"() -> (w306:u16)
    n160 = Index Array(array=w336) -> (element #1=w335:fxp<+/-,64,32>, element #2=w334:fxp<+/-,64,32>, element #3=w333:fxp<+/-,64,32>, element #4=w332:fxp<+/-,64,32>, element #5=w331:fxp<+/-,64,32>)  [unwired: 5 in]
    n161 = Index Array(array=w330) -> (element #1=w329:bool, element #2=w328:bool, element #3=w327:bool, element #4=w326:bool, element #5=w325:bool)  [unwired: 5 in]
    n162 = call "nism.step.p.fxp(modified).vi"("calls per sample"=w306, "reset"=w329, "minimum pulse"="minimum pulse", "position setpoint"=w335) -> ("steps generated"=w311:i32, "step"=w323:bool, "direction"=w324:bool)  [unwired: 4 in, 1 out]
    n163 = call "nism.step.p.fxp(modified).vi"("calls per sample"=w306, "reset"=w328, "minimum pulse"="minimum pulse", "position setpoint"=w334) -> ("steps generated"=w310:i32, "step"=w321:bool, "direction"=w322:bool)  [unwired: 4 in, 1 out]
    n164 = call "nism.step.p.fxp(modified).vi"("calls per sample"=w306, "reset"=w327, "minimum pulse"="minimum pulse", "position setpoint"=w333) -> ("steps generated"=w309:i32, "step"=w319:bool, "direction"=w320:bool)  [unwired: 4 in, 1 out]
    n165 = call "nism.step.p.fxp(modified).vi"("calls per sample"=w306, "reset"=w326, "minimum pulse"="minimum pulse", "position setpoint"=w332) -> ("steps generated"=w308:i32, "step"=w317:bool, "direction"=w318:bool)  [unwired: 4 in, 1 out]
    n166 = call "nism.step.p.fxp(modified).vi"("calls per sample"=w306, "reset"=w325, "minimum pulse"="minimum pulse", "position setpoint"=w331) -> ("steps generated"=w307:i32, "step"=w315:bool, "direction"=w316:bool)  [unwired: 4 in, 1 out]
    n167 = shared-variable "RT CompactRIO Target\\User-Defined Variables\\Axis 1.Steps Generated"(w311) -> ()  [unwired: 1 in, 1 out]
    n168 = shared-variable "RT CompactRIO Target\\User-Defined Variables\\Axis 2.Steps Generated"(w310) -> ()  [unwired: 1 in, 1 out]
    n169 = shared-variable "RT CompactRIO Target\\User-Defined Variables\\Axis 3.Steps Generated"(w309) -> ()  [unwired: 1 in, 1 out]
    n170 = shared-variable "RT CompactRIO Target\\User-Defined Variables\\Axis 4.Steps Generated"(w308) -> ()  [unwired: 1 in, 1 out]
    n171 = shared-variable "RT CompactRIO Target\\User-Defined Variables\\Axis 5.Steps Generated"(w307) -> ()  [unwired: 1 in, 1 out]
    n172 = shared-variable "RT CompactRIO Target\\User-Defined Variables\\Axis 1.Position Feedback"(w311) -> ()  [unwired: 1 in, 1 out]
    n173 = shared-variable "RT CompactRIO Target\\User-Defined Variables\\Axis 2.Position Feedback"(w310) -> ()  [unwired: 1 in, 1 out]
    n174 = shared-variable "RT CompactRIO Target\\User-Defined Variables\\Axis 3.Position Feedback"(w309) -> ()  [unwired: 1 in, 1 out]
    n175 = shared-variable "RT CompactRIO Target\\User-Defined Variables\\Axis 4.Position Feedback"(w308) -> ()  [unwired: 1 in, 1 out]
    n176 = shared-variable "RT CompactRIO Target\\User-Defined Variables\\Axis 5.Position Feedback"(w307) -> ()  [unwired: 1 in, 1 out]
    n177 = case shown="True" "STEP or CW? (T=STEP)" {
      tunnel: w324 -> [w368 w388]
      tunnel: w323 -> [w367 w378]
      tunnel: w322 -> [w366 w386]
      tunnel: w321 -> [w365 w376]
      tunnel: w320 -> [w364 w384]
      tunnel: w319 -> [w363 w374]
      tunnel: w318 -> [w362 w382]
      tunnel: w317 -> [w361 w372]
      tunnel: w316 -> [w360 w380]
      tunnel: w315 -> [w359 w370]
      tunnel: "Invert direction?" -> [w348 w389]
      tunnel: [w358 w387] -> w305
      tunnel: [w357 w377] -> w304
      tunnel: [w356 w385] -> w303
      tunnel: [w355 w375] -> w302
      tunnel: [w354 w383] -> w301
      tunnel: [w353 w373] -> w300
      tunnel: [w352 w381] -> w299
      tunnel: [w351 w371] -> w298
      tunnel: [w350 w379] -> w296
      tunnel: [w349 w369] -> w295
      frame False {
        n178 = call "Step_Dir_to_CW_CCW.vi"("invert"=w348, "step"=w367, "direction"=w368) -> ("CCW"=w357:bool, "CW"=w358:bool)  [unwired: 7 in]
        n179 = call "Step_Dir_to_CW_CCW.vi"("invert"=w348, "step"=w365, "direction"=w366) -> ("CCW"=w355:bool, "CW"=w356:bool)  [unwired: 7 in]
        n180 = call "Step_Dir_to_CW_CCW.vi"("invert"=w348, "step"=w363, "direction"=w364) -> ("CCW"=w353:bool, "CW"=w354:bool)  [unwired: 7 in]
        n181 = call "Step_Dir_to_CW_CCW.vi"("invert"=w348, "step"=w361, "direction"=w362) -> ("CCW"=w351:bool, "CW"=w352:bool)  [unwired: 7 in]
        n182 = call "Step_Dir_to_CW_CCW.vi"("invert"=w348, "step"=w359, "direction"=w360) -> ("CCW"=w349:bool, "CW"=w350:bool)  [unwired: 7 in]
      }
      frame True {
        n183 = case shown="True" w389 {
          tunnel: w388 -> [w399 w414]
          tunnel: [w399 w413] -> w387
          tunnel: w386 -> [w397 w412]
          tunnel: [w397 w411] -> w385
          tunnel: w384 -> [w395 w410]
          tunnel: [w395 w409] -> w383
          tunnel: w382 -> [w393 w408]
          tunnel: [w393 w407] -> w381
          tunnel: w380 -> [w391 w406]
          tunnel: [w391 w405] -> w379
          tunnel: w378 -> [w398 w404]
          tunnel: [w398 w404] -> w377
          tunnel: w376 -> [w396 w403]
          tunnel: [w396 w403] -> w375
          tunnel: w374 -> [w394 w402]
          tunnel: [w394 w402] -> w373
          tunnel: w372 -> [w392 w401]
          tunnel: [w392 w401] -> w371
          tunnel: w370 -> [w390 w400]
          tunnel: [w390 w400] -> w369
          frame False {
          }
          frame True {
            n184 = Not(x=w414) -> (.not. x?=w413:bool)
            n185 = Not(x=w412) -> (.not. x?=w411:bool)
            n186 = Not(x=w410) -> (.not. x?=w409:bool)
            n187 = Not(x=w408) -> (.not. x?=w407:bool)
            n188 = Not(x=w406) -> (.not. x?=w405:bool)
          }
        }
      }
    }
    n189 = case shown="\"Sync with Sensor\"" "Axis 5 Mode" {
      tunnel: [w338 w347] -> w293
      tunnel: w295 -> [w338 _]
      tunnel: w296 -> [w339 _]
      tunnel: [w339 "Sensor Sync DIR"] -> w294
      frame "No Sync", Default {
      }
      frame "Sync with Sensor" {
        n190 = local read "Number of pulses (N)"() -> (w342:i32)
        n191 = local read "Reset Flag"() -> (w340:bool)
        n192 = To Unsigned Long Integer(number=w342) -> (unsigned 32bit integer=w341:u32)
        n193 = call "Custom Freq Multiplier 3.vi"("Number of pulses"=w341, "Reset"=w340) -> ("DO State"=w347:bool, "Toggle Iterations"=→"Toggle Iterations":u32, "Time elapsed (ticks)"=→"Time elapsed (ticks)":u32, "FIFO Read Timed Out?"=→"FIFO Read Timed Out?":bool)  [unwired: 6 in]
      }
    }
    n194 = xnode "FPGA I/O Node"("Mod1/DIO0"=w305, "Mod1/DIO1"=w304, "Mod1/DIO2"=w303, "Mod1/DIO3"=w302, "Mod1/DIO4"=w301, "Mod1/DIO5"=w300, "Mod1/DIO6"=w299, "Mod1/DIO7"=w298, "Mod2/DIO0"=w294, "Mod2/DIO1"=w293) -> ()  [unwired: 10 in, 10 out]
  }
  n195 = timed-loop "Synchronization Loop" {
    timing: w8 -> [_]
    timing-out: [_] -> w7
    stop <- FALSE stop-if-true
    n196 = xnode "FPGA I/O Node"() -> ("Scan Clock"=w421:bool)  [unwired: 1 in, 1 out]
    n197 = global read "Global FPGA.vi" "Sync Enable"() -> (w420:bool)
    n198 = Select(t="Sync Value", s="Sync Enable override?", f=w420) -> (s? t:f=w417:bool)
    n199 = call-poly <vilib>:"nism.scan.generateSyncScan.vi"("scan enable?"=w417, "scan clock"=w421) -> ("timer control"=w422:T9)  [unwired: 3 in]
    n200 = global write "Global FPGA.vi" "Timer Control"(w422) -> ()
  }
  n201 = timed-loop "Reset Monitoring Loop" {
    timing: w6 -> [_]
    timing-out: [_] -> w5
    stop <- FALSE stop-if-true
    n202 = global read "Global FPGA.vi" "Reset Pending"() -> (w428:bool[])
    n203 = xnode "FPGA I/O Node"() -> ("Scan Clock"=w427:bool)  [unwired: 1 in, 1 out]
    n204 = feedback-in #2(w427) -> ()
    n205 = feedback #2() -> (w426:bool)  [unwired: 1 in]
    n206 = Greater?(x=w427, y=w426) -> (0:w432:bool)
    n207 = feedback #3() -> (w431:bool[])  [unwired: 1 in]
    n208 = Select(t=w428, s=w432, f=w431) -> (s? t:f=w429:bool[])
    n209 = feedback-in #3(w429) -> ()
    n210 = global write "Global FPGA.vi" "Reset"(w429) -> ()
  }
  n211 = node-c288(w5) -> ()
  n212 = node-c288(w7) -> ()
  n213 = node-c288(w9) -> ()
